vi "UpdateFlagState.vi"(7 "LabVIEW Web Service Request":refnum<class "Web Request.lvclass">, 9 "Room":i32, 10 "FlagState":u32) -> (2 "FlagOut":string)   [LabVIEW 2015]
uses:
  <vilib>/wsapi/Web Request.lvclass
  TypeDef/RoomsActionEnum.ctl
panel:
  out "request variables":cluster{"Key":string[], "Value":string[]}
  out "postdata":string
  # "Use the Web Service Request input terminal to call the VIs on the Web Services palette. Do not remove it from the connector pane unless you don't need access to the palette."
  # "Each additional control wired to the connector pane will be available as an input in the URL. To include an indicator in terminal-mode output (the default setting), it must also be wired to the connector pane."
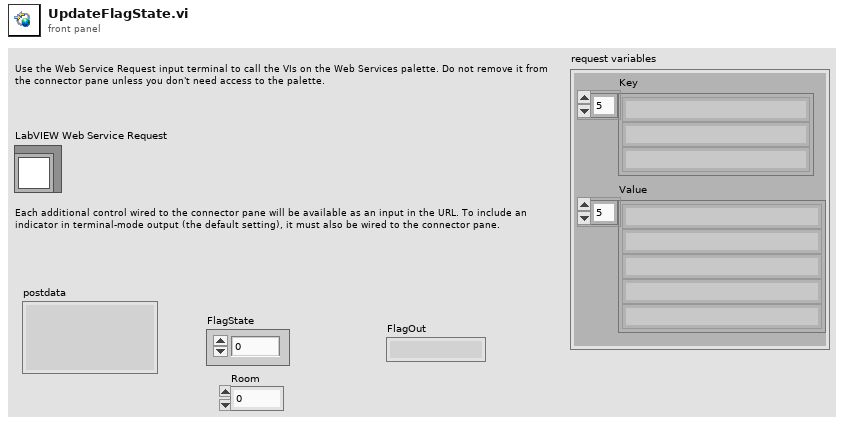
[diagram p1: front panel]
types:
  T1 = typedef "RoomsActionEnum.ctl" = enum16{"Init", "Add Room", "Remove Room", "Read Room", "Read Flag", "Read Flag State", "Write Flag State", "Read Flag Color", "Write Flag Color", "Read Bed Vacant", "Write Bed Vacant", "Read Personnel", "Add Personnel", "Remove Personnel", "Read Requests", "Add Request", "Remove Request", "Read Beacon ID", "Write Beacon ID", "Write Bed URL", "Read Bed URL", "Read Rooms Numbers", "Write Flag"}
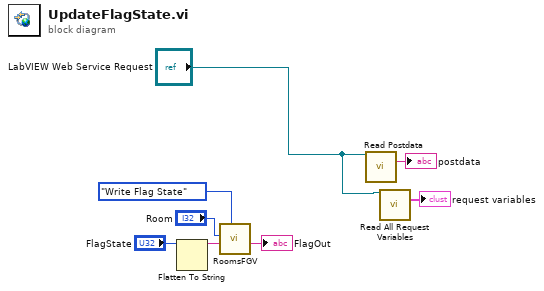
[diagram p0: block diagram]
diagram:
  n1 = Flatten To String(anything="FlagState") -> (data string=w5:string)  [unwired: 3 in, 2 out]
  n2 = call "RoomsFGV.vi"("Actions"=RoomsActionEnum."Write Flag State", "Data In"=w5, "Room"="Room") -> ("Data Out"=→"FlagOut":string)  [unwired: 7 in, 1 out]
  n3 = call <vilib>:"Read Postdata.vi"("LabVIEW Web Service Request"="LabVIEW Web Service Request") -> ("postdata"=→"postdata":string)  [unwired: 12 in, 2 out]
  n4 = call <vilib>:"Read All Request Variables.vi"("LabVIEW Web Service Request"="LabVIEW Web Service Request") -> ("request variables"=→"request variables":cluster{"Key":string[], "Value":string[]})  [unwired: 12 in, 2 out]
